vi "Add Lookup Event Listener Helper.vi"   [LabVIEW 2019, in "Lookup API.lvlib"]
doc: "<b>Description</b> A helper VI snippet for use with the Lookup API. Drop the contents of this VI directly onto your block diagram.\n\nAfter dropping this in your VI, follow the instructions in the labels to update the types."
uses:
  Lookup API.lvlib
  605cf116-c6a1-4699-92bc-2b46e486f691.vi
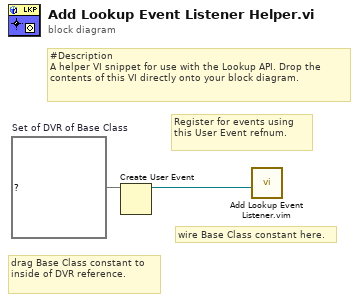
[diagram p0: block diagram]
diagram:
  w2 = set{refnum<data-value>} {}  # Set of DVR of Base Class
  # "Register for events using this User Event refnum."
  # "wire Base Class constant here."
  # "#Description\nA helper VI snippet for use with the Lookup API. Drop the contents of this VI directly onto your block diagram."
  # "drag Base Class constant to inside of DVR reference."
  n1 = Create User Event(user event datatype=w2) -> (user event=w1:refnum<user-event>)  [unwired: 1 in, 1 out]
  n2 = call "Add Lookup Event Listener.vim"("user event"=w1) -> ()  [unwired: 9 in, 2 out]
